vi "Load Effective Settings.vi"(8 "error in":errorcluster, 11 "Settings Service in":refnum<class "Settings Service.lvclass">) -> (0 "error out":errorcluster, 3 "Setting Service out":refnum<class "Settings Service.lvclass">)   [LabVIEW 2026, in "Settings Service.lvclass"]
uses:
  Settings Service.lvclass
  Settings Service.lvclass/Settings Service.ctl
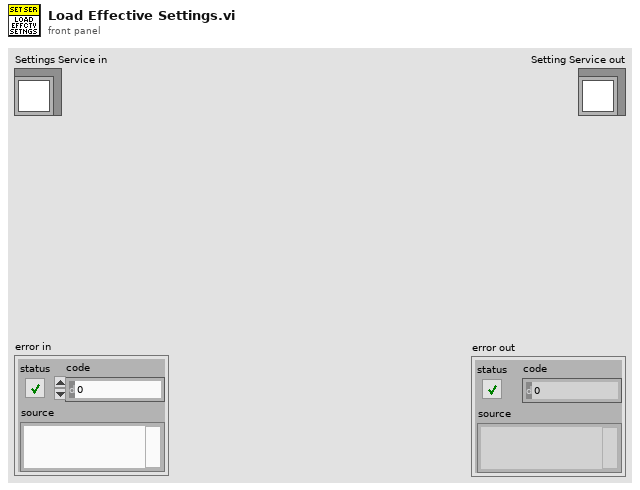
[diagram p1: front panel]
types:
  T1 = enum16{"open", "replace", "create", "open or create", "replace or create", "replace or create with confirmation"}
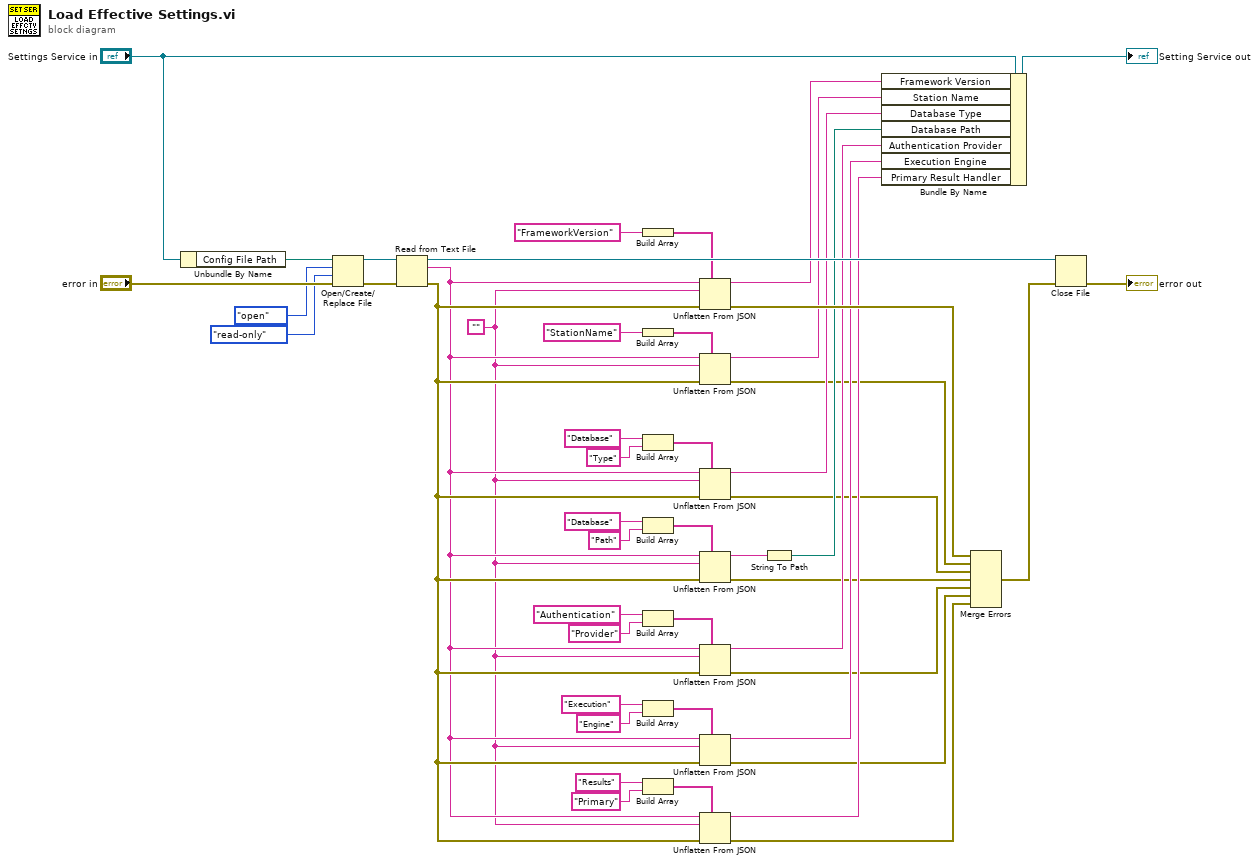
[diagram p0: block diagram]
diagram:
  w9 = ""
  n1 = Unbundle By Name("Settings Service in") -> ("Config File Path"=w1:path)
  n2 = Open/Create/Replace File(file path (use dialog)=w1, error in="error in", operation (0:open)=T1."open", access (0:read/write)=enum16{"read/write", "read-only", "write-only"}."read-only") -> (refnum out=w47:refnum<file>, error out=w44:errorcluster)  [unwired: 2 in, 1 out]
  n3 = Read from Text File(file (use dialog)=w47, error in=w44) -> (refnum out=w43:refnum<file>, text=w10:string, error out=w11:errorcluster)  [unwired: 2 in, 1 out]
  n4 = Build Array("FrameworkVersion") -> (w40:string[])
  n5 = Build Array("StationName") -> (w28:string[])
  n6 = Build Array("Database", "Type" ("element")) -> (w38:string[])
  n7 = Build Array("Database", "Path" ("element")) -> (w31:string[])
  n8 = Build Array("Authentication", "Provider" ("element")) -> (w21:string[])
  n9 = Build Array("Execution", "Engine" ("element")) -> (w17:string[])
  n10 = Build Array("Results", "Primary" ("element")) -> (w13:string[])
  n11 = Unflatten From JSON(path=w40, JSON string=w10, type and defaults=w9, error in (no error)=w11) -> (value=w29:string, error out=w36:errorcluster)  [unwired: 3 in]
  n12 = Unflatten From JSON(path=w28, JSON string=w10, type and defaults=w9, error in (no error)=w11) -> (value=w26:string, error out=w7:errorcluster)  [unwired: 3 in]
  n13 = Unflatten From JSON(path=w38, JSON string=w10, type and defaults=w9, error in (no error)=w11) -> (value=w25:string, error out=w6:errorcluster)  [unwired: 3 in]
  n14 = Unflatten From JSON(path=w31, JSON string=w10, type and defaults=w9, error in (no error)=w11) -> (value=w24:string, error out=w5:errorcluster)  [unwired: 3 in]
  n15 = Unflatten From JSON(path=w21, JSON string=w10, type and defaults=w9, error in (no error)=w11) -> (value=w19:string, error out=w4:errorcluster)  [unwired: 3 in]
  n16 = Unflatten From JSON(path=w17, JSON string=w10, type and defaults=w9, error in (no error)=w11) -> (value=w15:string, error out=w3:errorcluster)  [unwired: 3 in]
  n17 = Unflatten From JSON(path=w13, JSON string=w10, type and defaults=w9, error in (no error)=w11) -> (value=w8:string, error out=w2:errorcluster)  [unwired: 3 in]
  n18 = String To Path(string=w24) -> (path=w23:path)
  n19 = Bundle By Name(cluster="Settings Service in", "Framework Version"=w29, "Station Name"=w26, "Database Type"=w25, "Database Path"=w23, "Authentication Provider"=w19, "Execution Engine"=w15, "Primary Result Handler"=w8) -> (→"Setting Service out":refnum<class "Settings Service.lvclass">)
  n20 = Merge Errors(w36, w7, w6, w5, w4, w3, w2) -> (w35:errorcluster)
  n21 = Close File(refnum=w43, error in=w35) -> (error out=→"error out":errorcluster)  [unwired: 1 out]
